vi "GetSize2DMatrix.vi"(0 "Array IN (2D)":dbl[][](array[numeric])) -> (1 "# Cols":i32, 2 "# Rows":i32)   [LabVIEW 2017]
doc: "Get # of rows and columns in 2D array"
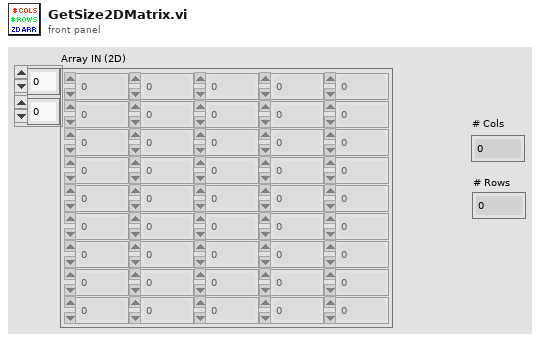
[diagram p1: front panel]
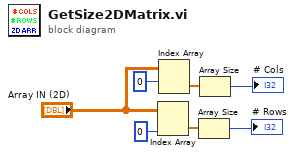
[diagram p0: block diagram]
diagram:
  n1 = Index Array(array="Array IN (2D)", index (col)=0 ("index (row)")) -> (element=w4:dbl[])  [unwired: 1 in]
  n2 = Index Array(array="Array IN (2D)", index (row)=0) -> (element=w6:dbl[])  [unwired: 1 in]
  n3 = Array Size(array=w4) -> (size(s)=→"# Rows":i32)
  n4 = Array Size(array=w6) -> (size(s)=→"# Cols":i32)
